vi "PrimaryInterfaceGetStartupData.vi"(8 "PrimaryInterface":refnum<k24>, 11 "error in":errorcluster) -> (0 "Startup data":T1, 3 "error out":errorcluster)   [LabVIEW 2023]
uses:
  C:/Users/fg/Documents/UniversalRobots.vi/UnderAutomation.UniversalRobots/lib/UnderAutomation.UniversalRobots.dll
  lib/UnderAutomation.UniversalRobots.dll
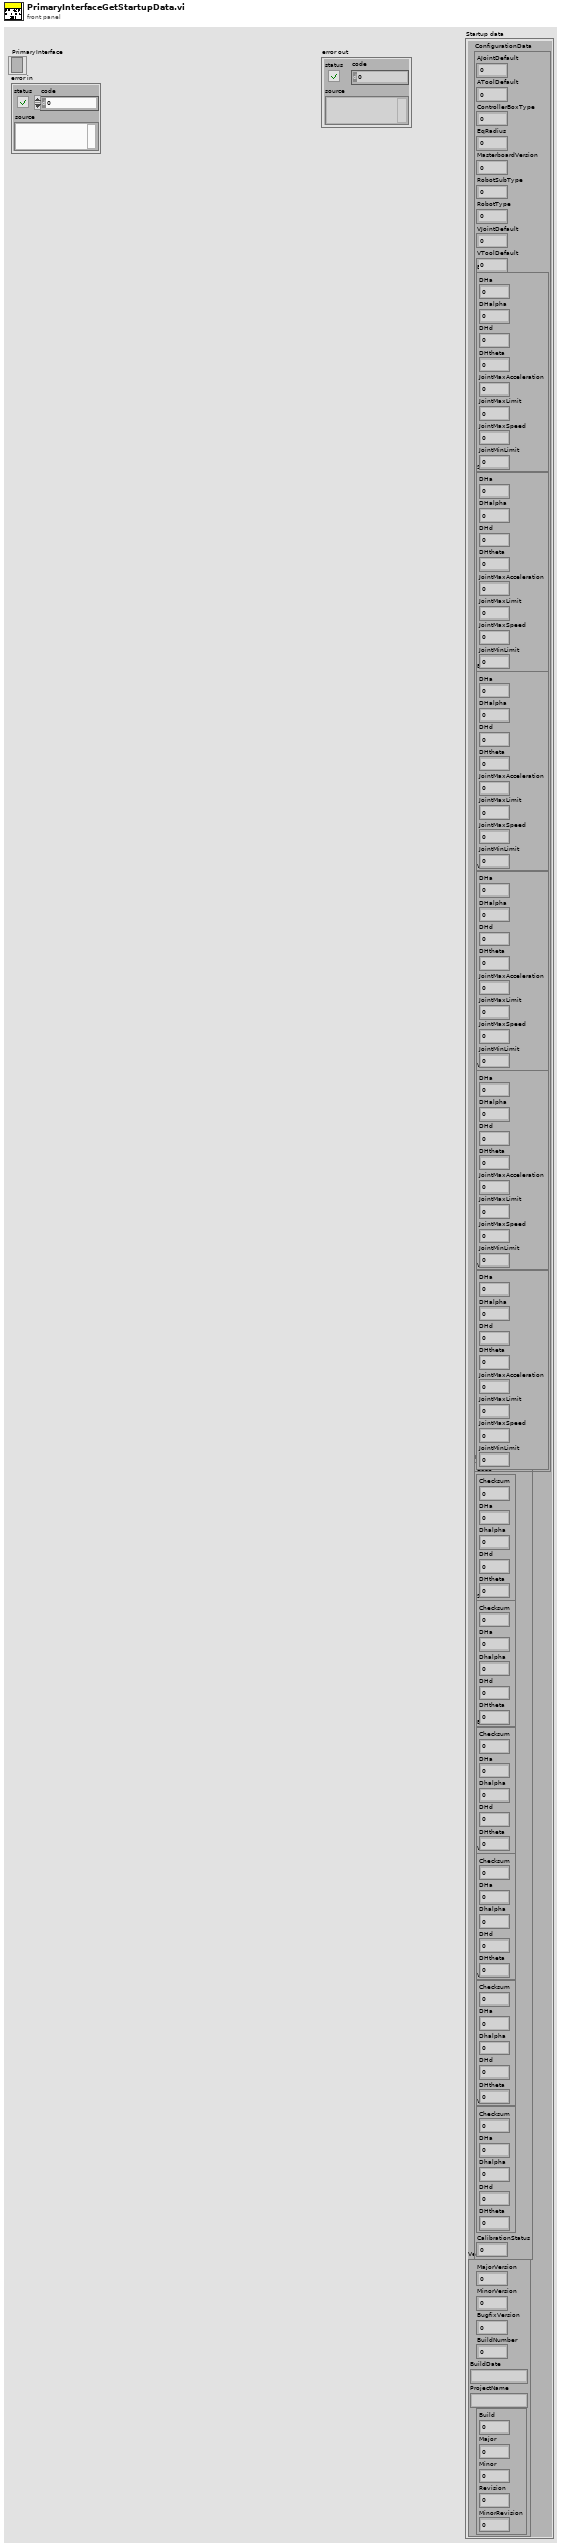
[diagram p1: front panel]
types:
  T1 = cluster{"ConfigurationData":cluster{"AJointDefault":dbl, "AToolDefault":dbl, "ControllerBoxType":i32, "EqRadius":dbl, "MasterboardVersion":i32, "RobotSubType":i32, "RobotType":i32, "VJointDefault":dbl, "VToolDefault":dbl, "Base":cluster{"DHa":dbl, "DHalpha":dbl, "DHd":dbl, "DHtheta":dbl, "JointMaxAcceleration":dbl, "JointMaxLimit":dbl, "JointMaxSpeed":dbl, "JointMinLimit":dbl}, "Shoulder":cluster{"DHa":dbl, "DHalpha":dbl, "DHd":dbl, "DHtheta":dbl, "JointMaxAcceleration":dbl, "JointMaxLimit":dbl, "JointMaxSpeed":dbl, "JointMinLimit":dbl}, "Elbow":cluster{"DHa":dbl, "DHalpha":dbl, "DHd":dbl, "DHtheta":dbl, "JointMaxAcceleration":dbl, "JointMaxLimit":dbl, "JointMaxSpeed":dbl, "JointMinLimit":dbl}, "Wrist1":cluster{"DHa":dbl, "DHalpha":dbl, "DHd":dbl, "DHtheta":dbl, "JointMaxAcceleration":dbl, "JointMaxLimit":dbl, "JointMaxSpeed":dbl, "JointMinLimit":dbl}, "Wrist2":cluster{"DHa":dbl, "DHalpha":dbl, "DHd":dbl, "DHtheta":dbl, "JointMaxAcceleration":dbl, "JointMaxLimit":dbl, "JointMaxSpeed":dbl, "JointMinLimit":dbl}, "Wrist3":cluster{"DHa":dbl, "DHalpha":dbl, "DHd":dbl, "DHtheta":dbl, "JointMaxAcceleration":dbl, "JointMaxLimit":dbl, "JointMaxSpeed":dbl, "JointMinLimit":dbl}}, "KinematicsInfo":cluster{"Base":cluster{"Checksum":i32, "DHa":dbl, "Dhalpha":dbl, "DHd":dbl, "DHtheta":dbl}, "Shoulder":cluster{"Checksum":i32, "DHa":dbl, "Dhalpha":dbl, "DHd":dbl, "DHtheta":dbl}, "Elbow":cluster{"Checksum":i32, "DHa":dbl, "Dhalpha":dbl, "DHd":dbl, "DHtheta":dbl}, "Wrist1":cluster{"Checksum":i32, "DHa":dbl, "Dhalpha":dbl, "DHd":dbl, "DHtheta":dbl}, "Wrist2":cluster{"Checksum":i32, "DHa":dbl, "Dhalpha":dbl, "DHd":dbl, "DHtheta":dbl}, "Wrist3":cluster{"Checksum":i32, "DHa":dbl, "Dhalpha":dbl, "DHd":dbl, "DHtheta":dbl}, "CalibrationStatus":i32}, "Version":cluster{"MajorVersion":u8, "MinorVersion":u8, "BugfixVersion":i32, "BuildNumber":i32, "BuildDate":string, "ProjectName":string, "Version":cluster{"Build":i32, "Major":i32, "Minor":i32, "Revision":i32, "MinorRevision":i16}}}
  T2 = cluster{"DHa":dbl, "DHalpha":dbl, "DHd":dbl, "DHtheta":dbl, "JointMaxAcceleration":dbl, "JointMaxLimit":dbl, "JointMaxSpeed":dbl, "JointMinLimit":dbl}
  T3 = cluster{"Checksum":i32, "DHa":dbl, "Dhalpha":dbl, "DHd":dbl, "DHtheta":dbl}
  T4 = cluster{"Build":i32, "Major":i32, "Minor":i32, "Revision":i32, "MinorRevision":i16}
  T5 = cluster{"AJointDefault":dbl, "AToolDefault":dbl, "ControllerBoxType":i32, "EqRadius":dbl, "MasterboardVersion":i32, "RobotSubType":i32, "RobotType":i32, "VJointDefault":dbl, "VToolDefault":dbl, cluster{"DHa":dbl, "DHalpha":dbl, "DHd":dbl, "DHtheta":dbl, "JointMaxAcceleration":dbl, "JointMaxLimit":dbl, "JointMaxSpeed":dbl, "JointMinLimit":dbl}, cluster{"DHa":dbl, "DHalpha":dbl, "DHd":dbl, "DHtheta":dbl, "JointMaxAcceleration":dbl, "JointMaxLimit":dbl, "JointMaxSpeed":dbl, "JointMinLimit":dbl}, cluster{"DHa":dbl, "DHalpha":dbl, "DHd":dbl, "DHtheta":dbl, "JointMaxAcceleration":dbl, "JointMaxLimit":dbl, "JointMaxSpeed":dbl, "JointMinLimit":dbl}, cluster{"DHa":dbl, "DHalpha":dbl, "DHd":dbl, "DHtheta":dbl, "JointMaxAcceleration":dbl, "JointMaxLimit":dbl, "JointMaxSpeed":dbl, "JointMinLimit":dbl}, cluster{"DHa":dbl, "DHalpha":dbl, "DHd":dbl, "DHtheta":dbl, "JointMaxAcceleration":dbl, "JointMaxLimit":dbl, "JointMaxSpeed":dbl, "JointMinLimit":dbl}, cluster{"DHa":dbl, "DHalpha":dbl, "DHd":dbl, "DHtheta":dbl, "JointMaxAcceleration":dbl, "JointMaxLimit":dbl, "JointMaxSpeed":dbl, "JointMinLimit":dbl}}
  T6 = cluster{cluster{"Checksum":i32, "DHa":dbl, "Dhalpha":dbl, "DHd":dbl, "DHtheta":dbl}, cluster{"Checksum":i32, "DHa":dbl, "Dhalpha":dbl, "DHd":dbl, "DHtheta":dbl}, cluster{"Checksum":i32, "DHa":dbl, "Dhalpha":dbl, "DHd":dbl, "DHtheta":dbl}, cluster{"Checksum":i32, "DHa":dbl, "Dhalpha":dbl, "DHd":dbl, "DHtheta":dbl}, cluster{"Checksum":i32, "DHa":dbl, "Dhalpha":dbl, "DHd":dbl, "DHtheta":dbl}, cluster{"Checksum":i32, "DHa":dbl, "Dhalpha":dbl, "DHd":dbl, "DHtheta":dbl}, "CalibrationStatus":i32}
  T7 = cluster{"MajorVersion":u8, "MinorVersion":u8, "BugfixVersion":i32, "BuildNumber":i32, "BuildDate":string, "ProjectName":string, cluster{"Build":i32, "Major":i32, "Minor":i32, "Revision":i32, "MinorRevision":i16}}
  T8 = cluster{cluster{"AJointDefault":dbl, "AToolDefault":dbl, "ControllerBoxType":i32, "EqRadius":dbl, "MasterboardVersion":i32, "RobotSubType":i32, "RobotType":i32, "VJointDefault":dbl, "VToolDefault":dbl, cluster{"DHa":dbl, "DHalpha":dbl, "DHd":dbl, "DHtheta":dbl, "JointMaxAcceleration":dbl, "JointMaxLimit":dbl, "JointMaxSpeed":dbl, "JointMinLimit":dbl}, cluster{"DHa":dbl, "DHalpha":dbl, "DHd":dbl, "DHtheta":dbl, "JointMaxAcceleration":dbl, "JointMaxLimit":dbl, "JointMaxSpeed":dbl, "JointMinLimit":dbl}, cluster{"DHa":dbl, "DHalpha":dbl, "DHd":dbl, "DHtheta":dbl, "JointMaxAcceleration":dbl, "JointMaxLimit":dbl, "JointMaxSpeed":dbl, "JointMinLimit":dbl}, cluster{"DHa":dbl, "DHalpha":dbl, "DHd":dbl, "DHtheta":dbl, "JointMaxAcceleration":dbl, "JointMaxLimit":dbl, "JointMaxSpeed":dbl, "JointMinLimit":dbl}, cluster{"DHa":dbl, "DHalpha":dbl, "DHd":dbl, "DHtheta":dbl, "JointMaxAcceleration":dbl, "JointMaxLimit":dbl, "JointMaxSpeed":dbl, "JointMinLimit":dbl}, cluster{"DHa":dbl, "DHalpha":dbl, "DHd":dbl, "DHtheta":dbl, "JointMaxAcceleration":dbl, "JointMaxLimit":dbl, "JointMaxSpeed":dbl, "JointMinLimit":dbl}}, cluster{cluster{"Checksum":i32, "DHa":dbl, "Dhalpha":dbl, "DHd":dbl, "DHtheta":dbl}, cluster{"Checksum":i32, "DHa":dbl, "Dhalpha":dbl, "DHd":dbl, "DHtheta":dbl}, cluster{"Checksum":i32, "DHa":dbl, "Dhalpha":dbl, "DHd":dbl, "DHtheta":dbl}, cluster{"Checksum":i32, "DHa":dbl, "Dhalpha":dbl, "DHd":dbl, "DHtheta":dbl}, cluster{"Checksum":i32, "DHa":dbl, "Dhalpha":dbl, "DHd":dbl, "DHtheta":dbl}, cluster{"Checksum":i32, "DHa":dbl, "Dhalpha":dbl, "DHd":dbl, "DHtheta":dbl}, "CalibrationStatus":i32}, cluster{"MajorVersion":u8, "MinorVersion":u8, "BugfixVersion":i32, "BuildNumber":i32, "BuildDate":string, "ProjectName":string, cluster{"Build":i32, "Major":i32, "Minor":i32, "Revision":i32, "MinorRevision":i16}}}
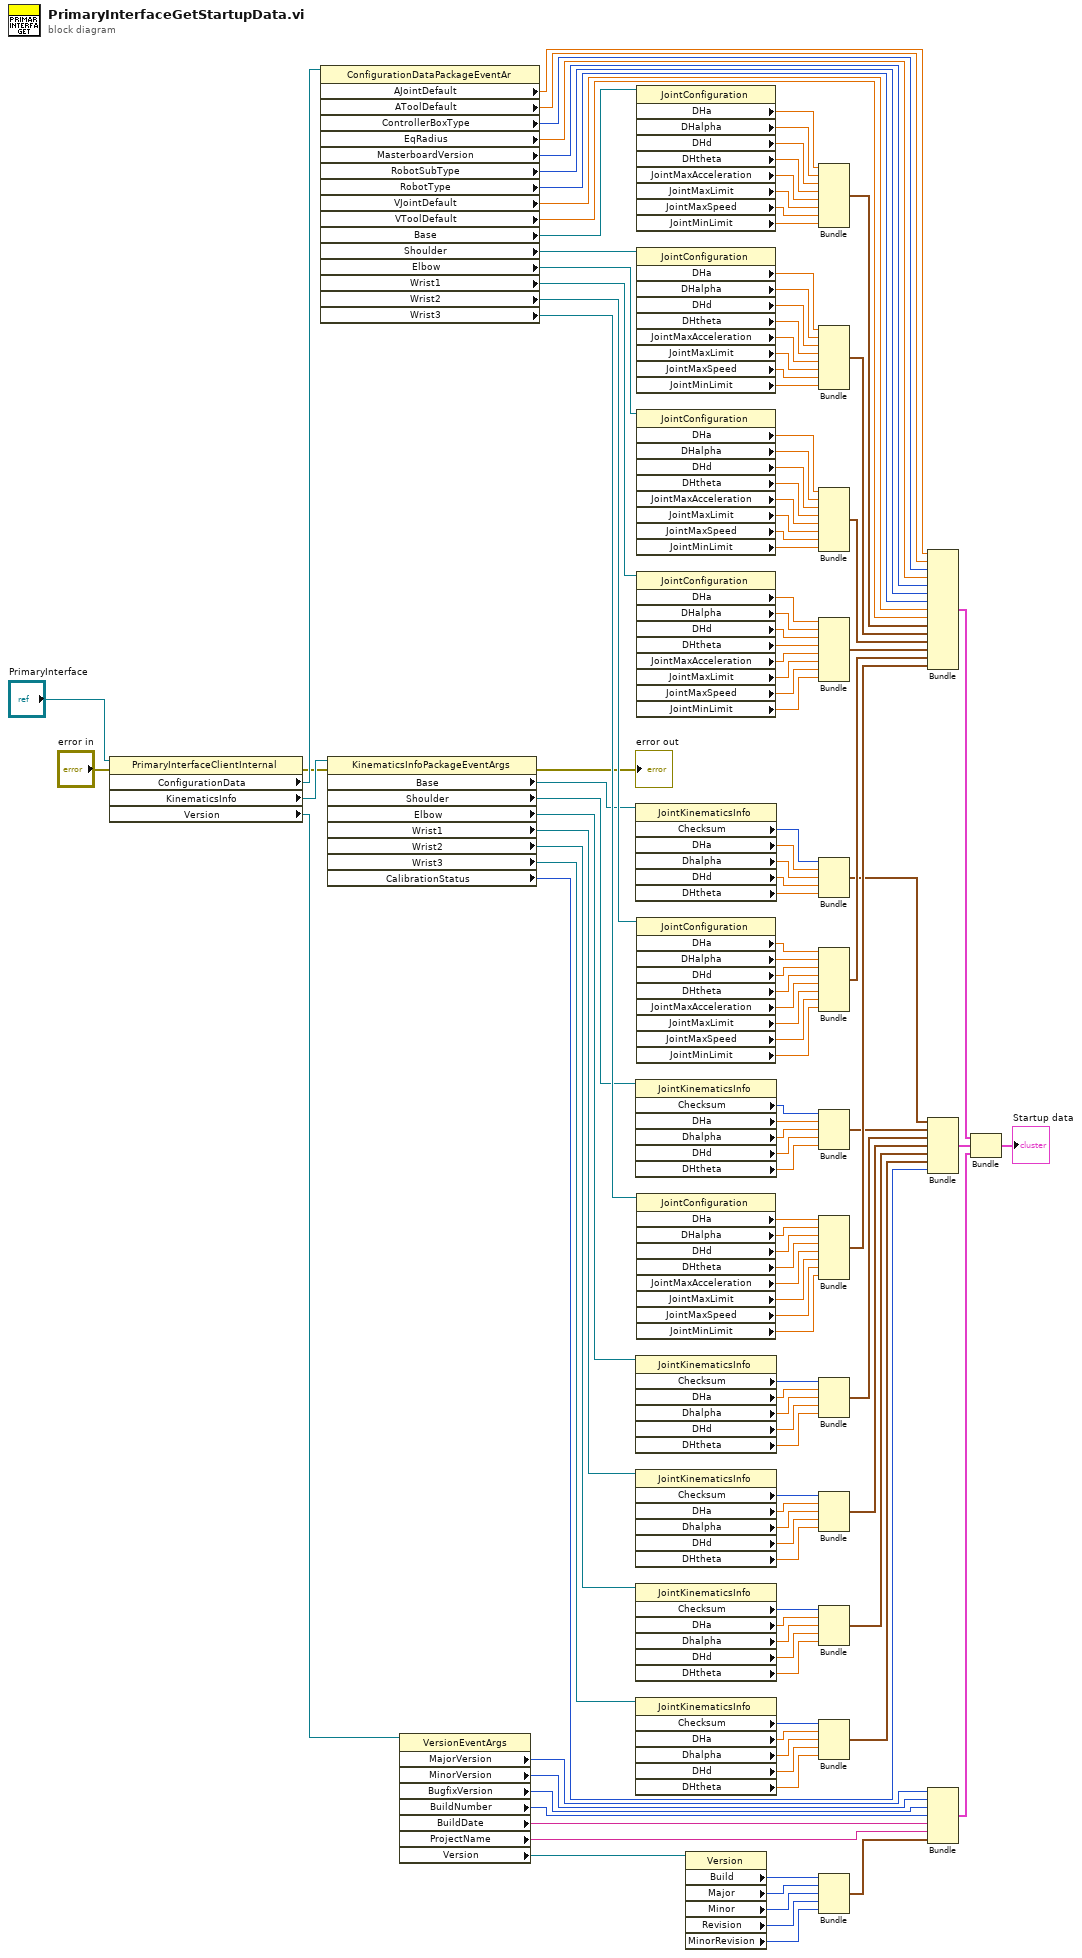
[diagram p0: block diagram]
diagram:
  n1 = property class="PrimaryInterfaceClientInternal"(reference="PrimaryInterface", error in="error in") -> (error out=w3:errorcluster, "ConfigurationData"=w135:refnum<k24>, "KinematicsInfo"=w65:refnum<k24>, "Version"=w21:refnum<k24>)  [unwired: 1 out]
  n2 = property class="ConfigurationDataPackageEventAr"(reference=w135) -> ("AJointDefault"=w80:dbl, "AToolDefault"=w79:dbl, "ControllerBoxType"=w78:i32, "EqRadius"=w77:dbl, "MasterboardVersion"=w76:i32, "RobotSubType"=w75:i32, "RobotType"=w74:i32, "VJointDefault"=w73:dbl, "VToolDefault"=w72:dbl, "Base"=w134:refnum<k24>, "Shoulder"=w85:refnum<k24>, "Elbow"=w84:refnum<k24>, "Wrist1"=w83:refnum<k24>, "Wrist2"=w82:refnum<k24>, "Wrist3"=w81:refnum<k24>)  [unwired: 1 in, 2 out]
  n3 = property class="KinematicsInfoPackageEventArgs"(reference=w65, error in=w3) -> (error out=→"error out":errorcluster, "Base"=w64:refnum<k24>, "Shoulder"=w33:refnum<k24>, "Elbow"=w32:refnum<k24>, "Wrist1"=w31:refnum<k24>, "Wrist2"=w30:refnum<k24>, "Wrist3"=w29:refnum<k24>, "CalibrationStatus"=w22:i32)  [unwired: 1 out]
  n4 = property class="VersionEventArgs"(reference=w21) -> ("MajorVersion"=w20:u8, "MinorVersion"=w19:u8, "BugfixVersion"=w18:i32, "BuildNumber"=w17:i32, "BuildDate"=w16:string, "ProjectName"=w15:string, "Version"=w14:refnum<k24>)  [unwired: 1 in, 2 out]
  n5 = property class="JointKinematicsInfo"(reference=w64) -> ("Checksum"=w63:i32, "DHa"=w62:dbl, "Dhalpha"=w61:dbl, "DHd"=w60:dbl, "DHtheta"=w59:dbl)  [unwired: 1 in, 2 out]
  n6 = property class="JointKinematicsInfo"(reference=w33) -> ("Checksum"=w54:i32, "DHa"=w55:dbl, "Dhalpha"=w56:dbl, "DHd"=w57:dbl, "DHtheta"=w58:dbl)  [unwired: 1 in, 2 out]
  n7 = property class="JointKinematicsInfo"(reference=w32) -> ("Checksum"=w53:i32, "DHa"=w52:dbl, "Dhalpha"=w51:dbl, "DHd"=w50:dbl, "DHtheta"=w49:dbl)  [unwired: 1 in, 2 out]
  n8 = property class="JointKinematicsInfo"(reference=w31) -> ("Checksum"=w44:i32, "DHa"=w45:dbl, "Dhalpha"=w46:dbl, "DHd"=w47:dbl, "DHtheta"=w48:dbl)  [unwired: 1 in, 2 out]
  n9 = property class="JointKinematicsInfo"(reference=w30) -> ("Checksum"=w43:i32, "DHa"=w42:dbl, "Dhalpha"=w41:dbl, "DHd"=w40:dbl, "DHtheta"=w39:dbl)  [unwired: 1 in, 2 out]
  n10 = property class="JointKinematicsInfo"(reference=w29) -> ("Checksum"=w34:i32, "DHa"=w35:dbl, "Dhalpha"=w36:dbl, "DHd"=w37:dbl, "DHtheta"=w38:dbl)  [unwired: 1 in, 2 out]
  n11 = property class="JointConfiguration"(reference=w134) -> ("DHa"=w133:dbl, "DHalpha"=w132:dbl, "DHd"=w131:dbl, "DHtheta"=w129:dbl, "JointMaxAcceleration"=w130:dbl, "JointMaxLimit"=w128:dbl, "JointMaxSpeed"=w127:dbl, "JointMinLimit"=w126:dbl)  [unwired: 1 in, 2 out]
  n12 = property class="JointConfiguration"(reference=w85) -> ("DHa"=w86:dbl, "DHalpha"=w87:dbl, "DHd"=w88:dbl, "DHtheta"=w90:dbl, "JointMaxAcceleration"=w89:dbl, "JointMaxLimit"=w91:dbl, "JointMaxSpeed"=w92:dbl, "JointMinLimit"=w93:dbl)  [unwired: 1 in, 2 out]
  n13 = property class="JointConfiguration"(reference=w84) -> ("DHa"=w101:dbl, "DHalpha"=w100:dbl, "DHd"=w99:dbl, "DHtheta"=w97:dbl, "JointMaxAcceleration"=w98:dbl, "JointMaxLimit"=w96:dbl, "JointMaxSpeed"=w95:dbl, "JointMinLimit"=w94:dbl)  [unwired: 1 in, 2 out]
  n14 = property class="JointConfiguration"(reference=w83) -> ("DHa"=w118:dbl, "DHalpha"=w119:dbl, "DHd"=w120:dbl, "DHtheta"=w122:dbl, "JointMaxAcceleration"=w121:dbl, "JointMaxLimit"=w123:dbl, "JointMaxSpeed"=w124:dbl, "JointMinLimit"=w125:dbl)  [unwired: 1 in, 2 out]
  n15 = property class="JointConfiguration"(reference=w82) -> ("DHa"=w117:dbl, "DHalpha"=w116:dbl, "DHd"=w115:dbl, "DHtheta"=w113:dbl, "JointMaxAcceleration"=w114:dbl, "JointMaxLimit"=w112:dbl, "JointMaxSpeed"=w111:dbl, "JointMinLimit"=w110:dbl)  [unwired: 1 in, 2 out]
  n16 = property class="JointConfiguration"(reference=w81) -> ("DHa"=w102:dbl, "DHalpha"=w103:dbl, "DHd"=w104:dbl, "DHtheta"=w106:dbl, "JointMaxAcceleration"=w105:dbl, "JointMaxLimit"=w107:dbl, "JointMaxSpeed"=w108:dbl, "JointMinLimit"=w109:dbl)  [unwired: 1 in, 2 out]
  n17 = property class="Version"(reference=w14) -> ("Build"=w13:i32, "Major"=w12:i32, "Minor"=w11:i32, "Revision"=w10:i32, "MinorRevision"=w9:i16)  [unwired: 1 in, 2 out]
  n18 = Bundle("DHa"=w133, "DHalpha"=w132, "DHd"=w131, "DHtheta"=w129, "JointMaxAcceleration"=w130, "JointMaxLimit"=w128, "JointMaxSpeed"=w127, "JointMinLimit"=w126) -> (w71:T2)  [unwired: 1 in]
  n19 = Bundle("DHa"=w86, "DHalpha"=w87, "DHd"=w88, "DHtheta"=w90, "JointMaxAcceleration"=w89, "JointMaxLimit"=w91, "JointMaxSpeed"=w92, "JointMinLimit"=w93) -> (w70:T2)  [unwired: 1 in]
  n20 = Bundle("DHa"=w101, "DHalpha"=w100, "DHd"=w99, "DHtheta"=w97, "JointMaxAcceleration"=w98, "JointMaxLimit"=w96, "JointMaxSpeed"=w95, "JointMinLimit"=w94) -> (w69:T2)  [unwired: 1 in]
  n21 = Bundle("DHa"=w118, "DHalpha"=w119, "DHd"=w120, "DHtheta"=w122, "JointMaxAcceleration"=w121, "JointMaxLimit"=w123, "JointMaxSpeed"=w124, "JointMinLimit"=w125) -> (w68:T2)  [unwired: 1 in]
  n22 = Bundle("Checksum"=w63, "DHa"=w62, "Dhalpha"=w61, "DHd"=w60, "DHtheta"=w59) -> (w28:T3)  [unwired: 1 in]
  n23 = Bundle("DHa"=w117, "DHalpha"=w116, "DHd"=w115, "DHtheta"=w113, "JointMaxAcceleration"=w114, "JointMaxLimit"=w112, "JointMaxSpeed"=w111, "JointMinLimit"=w110) -> (w67:T2)  [unwired: 1 in]
  n24 = Bundle("Checksum"=w54, "DHa"=w55, "Dhalpha"=w56, "DHd"=w57, "DHtheta"=w58) -> (w27:T3)  [unwired: 1 in]
  n25 = Bundle("DHa"=w102, "DHalpha"=w103, "DHd"=w104, "DHtheta"=w106, "JointMaxAcceleration"=w105, "JointMaxLimit"=w107, "JointMaxSpeed"=w108, "JointMinLimit"=w109) -> (w66:T2)  [unwired: 1 in]
  n26 = Bundle("Checksum"=w53, "DHa"=w52, "Dhalpha"=w51, "DHd"=w50, "DHtheta"=w49) -> (w26:T3)  [unwired: 1 in]
  n27 = Bundle("Checksum"=w44, "DHa"=w45, "Dhalpha"=w46, "DHd"=w47, "DHtheta"=w48) -> (w25:T3)  [unwired: 1 in]
  n28 = Bundle("Checksum"=w43, "DHa"=w42, "Dhalpha"=w41, "DHd"=w40, "DHtheta"=w39) -> (w24:T3)  [unwired: 1 in]
  n29 = Bundle("Checksum"=w34, "DHa"=w35, "Dhalpha"=w36, "DHd"=w37, "DHtheta"=w38) -> (w23:T3)  [unwired: 1 in]
  n30 = Bundle("Build"=w13, "Major"=w12, "Minor"=w11, "Revision"=w10, "MinorRevision"=w9) -> (w8:T4)  [unwired: 1 in]
  n31 = Bundle("AJointDefault"=w80, "AToolDefault"=w79, "ControllerBoxType"=w78, "EqRadius"=w77, "MasterboardVersion"=w76, "RobotSubType"=w75, "RobotType"=w74, "VJointDefault"=w73, "VToolDefault"=w72, w71, w70, w69, w68, w67, w66) -> (w5:T5)  [unwired: 1 in]
  n32 = Bundle(w28, w27, w26, w25, w24, w23, "CalibrationStatus"=w22) -> (w6:T6)  [unwired: 1 in]
  n33 = Bundle("MajorVersion"=w20, "MinorVersion"=w19, "BugfixVersion"=w18, "BuildNumber"=w17, "BuildDate"=w16, "ProjectName"=w15, w8) -> (w7:T7)  [unwired: 1 in]
  n34 = Bundle(w5, w6, w7) -> (→"Startup data":T8)  [unwired: 1 in]
